vi "Filter Boolean Input by Time.vi"(7 "Delay (2 s)":dbl=2.0, 11 "Boolean In":bool) -> (3 "Boolean Out":bool)   [LabVIEW 2013]
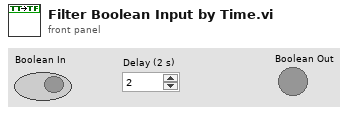
[diagram p1: front panel]
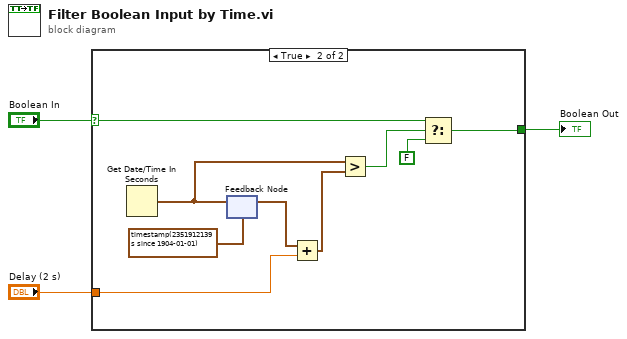
[diagram p0: block diagram]
diagram:
  n1 = case shown="True" "Boolean In" {
    selector: "Boolean In" -> [w4 w6]
    tunnel: [w4 w8] -> w3
    tunnel: "Delay (2 s)" -> [_ w5]
    frame False {
    }
    frame True {
      n2 = Get Date/Time In Seconds() -> (seconds since 1Jan1904=w11:timestamp)
      n3 = feedback #1(timestamp(2351912139.1919804 s since 1904-01-01) ("seconds since 1Jan1904")) -> (w13:timestamp)
      n4 = feedback-in #1(w11) -> ()
      n5 = Add(x=w13, y=w5) -> (x+y=w12:timestamp)
      n6 = Greater?(x=w11, y=w12) -> (0:w10:bool)
      n7 = Select(t=w6, s=w10, f=FALSE) -> (s? t:f=w8:bool)
    }
  }
  "Boolean Out" <- w3
